vi "get waveform - voltage range scaled.vi"(8 "error in (no error)":errorcluster caption="에러 입력(에러 없음)", 11 "Waveform Obj 입력":refnum<class "Waveform Obj.lvclass">) -> (0 "error out":errorcluster caption="에러 출력", 2 "scaled waveform":waveform(dbl), 3 "Waveform Obj 출력":refnum<class "Waveform Obj.lvclass">)   [LabVIEW 2020, in "Waveform Obj.lvclass"]
uses:
  Waveform Obj.lvclass
  Waveform Obj.lvclass/Waveform Obj.ctl
  Accessors/Read voltage range.vi
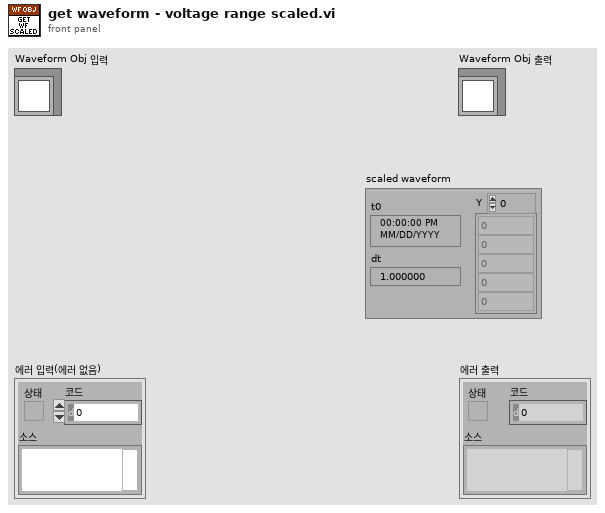
[diagram p1: front panel]
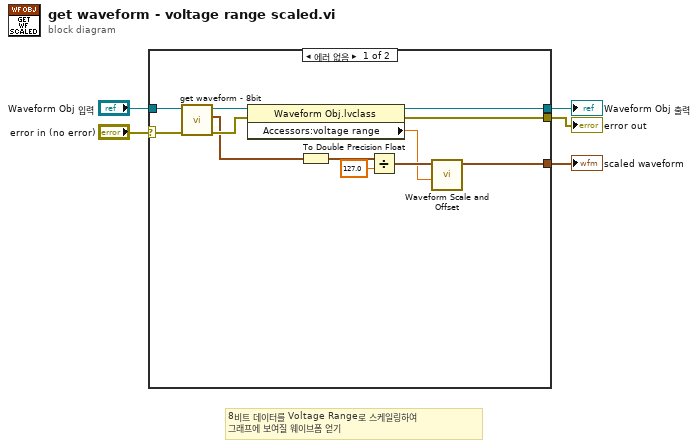
[diagram p0: block diagram]
diagram:
  # "8비트 데이터를 Voltage Range로 스케일링하여\n그래프에 보여질 웨이브폼 얻기"
  n1 = case shown="에러 없음" "error in (no error)" {
    selector: "error in (no error)" -> [w17 w19]
    tunnel: [w12 w19] -> w3
    tunnel: [w11 w18] -> w4
    tunnel: "Waveform Obj 입력" -> [w8 w18]
    tunnel: [w13 _] -> w1
    frame No Error {
      n2 = call-dynamic "get waveform - 8bit.vi"("error in (no error)"=w17, "Waveform Obj 입력"=w8) -> ("error out"=w9:errorcluster, "8bit waveform"=w6:waveform(i8), "Waveform Obj 출력"=w7:refnum<class "Waveform Obj.lvclass">)  [unwired: 6 in, 1 out]
      n3 = property class="Waveform Obj.lvclass"(reference=w7, error in=w9) -> (reference out=w11:refnum<class "Waveform Obj.lvclass">, error out=w12:errorcluster, "Accessors:voltage range"=w10:dbl)
      n4 = To Double Precision Float(number=w6) -> (double precision float=w16:waveform(dbl))
      n5 = Divide(x=w16, y=127.0) -> (x/y=w14:waveform(dbl))
      n6 = call <vilib>:"Waveform Scale and Offset.vi"("scale"=w10, "waveform in"=w14) -> ("waveform out"=w13:waveform(dbl))  [unwired: 8 in, 1 out]
    }
    frame Error {
    }
  }
  "error out" <- w3
  "Waveform Obj 출력" <- w4
  "scaled waveform" <- w1
